vi "Queue Write.vi"(8 "Error in (no error)":errorcluster caption="error out（no error）", 9 "Group Count":i32, 10 "Input Array":dbl[][](array[numeric]), 11 "Queue Input":refnum<queue>) -> (0 "Error out":errorcluster caption="error out", 3 "Queue output":refnum<queue>)   [LabVIEW 2019]
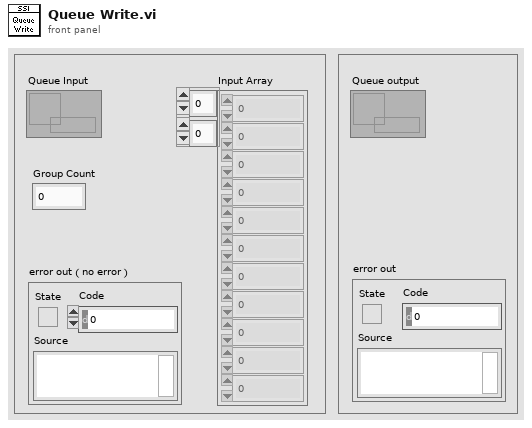
[diagram p1: front panel]
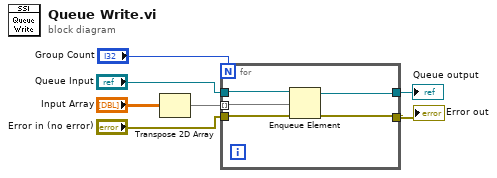
[diagram p0: block diagram]
diagram:
  n1 = Transpose 2D Array(2D array="Input Array") -> (transposed array=w7:dbl[][])
  n2 = for {
    N: "Group Count" -> [_]
    tunnel: "Queue Input" -> [w12]
    tunnel: "Error in (no error)" -> [w11]
    tunnel: w7 -> [w10] mode=indexing
    tunnel: [w8] -> w3
    tunnel: [w9] -> w2
    n3 = Enqueue Element(queue=w12, element=w10, error in (no error)=w11) -> (queue out=w9:refnum<queue>, error out=w8:errorcluster)  [unwired: 1 in, 1 out]
  }
  "Error out" <- w3
  "Queue output" <- w2
